vi "Test Filter.vi"() -> ()   [LabVIEW 2021]
uses:
  <vilib>/CIF Foundation/CIF Enet Parse and Build/typedef/L2 & L3/L2-L3 Packet  Addressing.ctl
  <vilib>/CIF Foundation/CIF Enet Parse and Build/typedef/L2 & L3/Packet Type.ctl
  <vilib>/CIF Foundation/CIF Enet Parse and Build/typedef/L2 & L3/IPV4 Filter.ctl
  <vilib>/CIF Foundation/CIF Enet Parse and Build/typedef/L2 & L3/IPV4 Protocol Ring.ctl
  <vilib>/CIF Foundation/CIF Enet Parse and Build/typedef/L2 & L3/L2 Filter.ctl
  L2ENET_RW_XNET/src/typedef/trash_Filter.ctl
  L2ENET_RW_CORE.lvclass/L2ENET_RW_CORE.ctl
  Accessors/Write Filter.vi
  <vilib>/CIF Foundation/CIF Utilities/Networking/IPV4/Calculate IP Header Checksum.vi
  <vilib>/CIF Foundation/CIF Enet Parse and Build/Packet Parse and Build/Packet Create L2&L3/Worker SubVIs/Create UDP Pseudoheader.vi
  <vilib>/CIF Foundation/CIF Enet Parse and Build/Packet Parse and Build/Packet Create L2&L3/Create UDP Header.vi
  <vilib>/CIF Foundation/CIF Enet Parse and Build/Packet Parse and Build/Packet Create L2&L3/Create IPV4 Header.vi
  <vilib>/CIF Foundation/CIF Enet Parse and Build/Packet Parse and Build/Packet Create L2&L3/Create L2 Header.vi
  <vilib>/CIF Foundation/CIF Enet Parse and Build/Packet Parse and Build/Filter and Parse L2&L3/Filter.vi
  <vilib>/CIF Foundation/CIF Utilities/DataTypes/Flatten Unflatten/Flatten U32.vi
  <vilib>/CIF Foundation/CIF Utilities/DataTypes/Flatten Unflatten/Flatten U16.vi
  <vilib>/CIF Foundation/CIF Utilities/DataTypes/Split Join/Join U8.vi
  <vilib>/CIF Foundation/CIF Utilities/DataTypes/Split Join/Join U16.vi
  <vilib>/CIF Foundation/CIF Enet Parse and Build/Packet Parse and Build/Packet Create L2&L3/Worker SubVIs/Create VLAN Tag.vi
  <vilib>/CIF Foundation/CIF Enet Parse and Build/Packet Parse and Build/Utilities/Create Multicast MAC Address.vi
  <vilib>/CIF Foundation/CIF Utilities/Networking/IPV4/Check Multicast IP.vi
  <vilib>/CIF Foundation/CIF Enet Parse and Build/Packet Parse and Build/Filter and Parse L2&L3/Parse L2 Header.vi
  <vilib>/CIF Foundation/CIF Enet Parse and Build/Packet Parse and Build/Filter and Parse L2&L3/Parse IPV4 Header.vi
  <vilib>/CIF Foundation/CIF Enet Parse and Build/Packet Parse and Build/Filter and Parse L2&L3/Parse UDP Header.vi
  <vilib>/CIF Foundation/CIF Enet Parse and Build/Packet Parse and Build/Filter and Parse L2&L3/Parse TCP Header.vi
  <vilib>/CIF Foundation/CIF Utilities/DataTypes/Flatten Unflatten/Unflatten U16.vi
  <vilib>/CIF Foundation/CIF Utilities/DataTypes/Split Join/Split U8.vi
  <vilib>/CIF Foundation/CIF Utilities/DataTypes/Flatten Unflatten/Unflatten U32.vi
  <vilib>/CIF Foundation/CIF Utilities/DataTypes/Split Join/Split U16.vi
  L2ENET_RW_CORE.lvclass
  <vilib>/CIF Foundation/CIF Enet Parse and Build/Ethernet_Parse_Build_CIF.lvlib
panel:
  out "Pass":bool
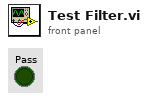
[diagram p1: front panel]
types:
  T1 = typedef "trash_Filter.ctl" = cluster{"L2 Filter":T2, "IPV4 Filter":T3}
  T2 = typedef "Ethernet_Parse_Build_CIF.lvlib/L2 Filter.ctl" = cluster{"DMAC Filter":bool, "DMAC":u8[], "SMAC Filter":bool, "SMAC":u8[], "EtherType Filter":bool, "EtherType":u16, "VLAN Filter":bool, "VLAN":u16, "PCP Filter":bool, "PCP":u8}
  T3 = typedef "Ethernet_Parse_Build_CIF.lvlib/IPV4 Filter.ctl" = cluster{"Source IP Filter":bool, "Source IP Address":u32, "Destination  IP Filter":bool, "Dest IP Address":u32, "IP Protocol Filter":bool, "Protocol":T4, "Source Port Filter":bool, "Source Port":u16, "Dest Port Filter ":bool, "Dest Port":u16}
  T4 = typedef "Ethernet_Parse_Build_CIF.lvlib/IPV4 Protocol Ring.ctl" = u8
  T5 = typedef "Ethernet_Parse_Build_CIF.lvlib/L2-L3 Packet  Addressing.ctl" = cluster{"Dest MAC Address":u8[], "Source MAC Address":u8[], "Packet Type":T6, "Ethertype":u16, "Source IP Address":u32, "Dest IP Address":u32, "DST Port":u16, "SRC Port":u16, "VLAN Tagged?":bool, "VLAN":u16, "PCP":u8}
  T6 = typedef "Ethernet_Parse_Build_CIF.lvlib/Packet Type.ctl" = enum16{"RAW", "UDP"}
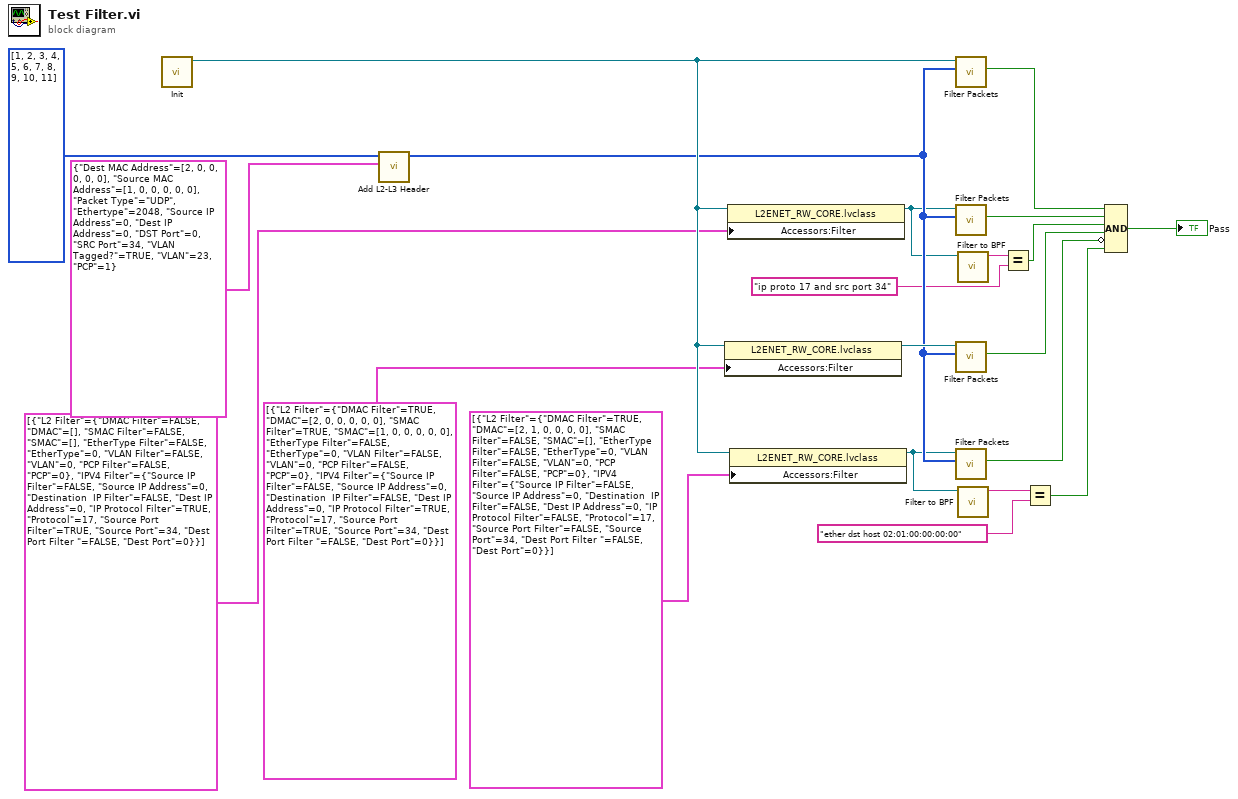
[diagram p0: block diagram]
diagram:
  n1 = call "Init.vi"() -> ("L2Enet_RW_CORE out"=w19:refnum<class "L2ENET_RW_CORE.lvclass">)  [unwired: 10 in, 1 out]
  n2 = call <vilib>:"Add L2-L3 Header.vi"("Addressing"=T5 {"Dest MAC Address"=[2, 0, 0, 0, 0, 0], "Source MAC Address"=[1, 0, 0, 0, 0, 0], "Packet Type"=enum."UDP", "Ethertype"=2048, "Source IP Address"=0, "Dest IP Address"=0, "DST Port"=0, "SRC Port"=34, "VLAN Tagged?"=TRUE, "VLAN"=23, "PCP"=1}, "Payload (bytes)"=u8[] [1, 2, 3, 4, 5, 6, 7, 8, 9, 10, 11]) -> ("Packet Data Out"=w12:u8[])  [unwired: 9 in]
  n3 = property class="L2ENET_RW_CORE.lvclass"(reference=w19, "Accessors:Filter"=T1[] [{"L2 Filter"={"DMAC Filter"=TRUE, "DMAC"=[2, 0, 0, 0, 0, 0], "SMAC Filter"=TRUE, "SMAC"=[1, 0, 0, 0, 0, 0], "EtherType Filter"=FALSE, "EtherType"=0, "VLAN Filter"=FALSE, "VLAN"=0, "PCP Filter"=FALSE, "PCP"=0}, "IPV4 Filter"={"Source IP Filter"=FALSE, "Source IP Address"=0, "Destination  IP Filter"=FALSE, "Dest IP Address"=0, "IP Protocol Filter"=TRUE, "Protocol"=17, "Source Port Filter"=TRUE, "Source Port"=34, "Dest Port Filter "=FALSE, "Dest Port"=0}}] ("Filter")) -> (reference out=w18:refnum<class "L2ENET_RW_CORE.lvclass">)  [unwired: 1 in, 1 out]
  n4 = property class="L2ENET_RW_CORE.lvclass"(reference=w19, "Accessors:Filter"=T1[] [{"L2 Filter"={"DMAC Filter"=FALSE, "DMAC"=[], "SMAC Filter"=FALSE, "SMAC"=[], "EtherType Filter"=FALSE, "EtherType"=0, "VLAN Filter"=FALSE, "VLAN"=0, "PCP Filter"=FALSE, "PCP"=0}, "IPV4 Filter"={"Source IP Filter"=FALSE, "Source IP Address"=0, "Destination  IP Filter"=FALSE, "Dest IP Address"=0, "IP Protocol Filter"=TRUE, "Protocol"=17, "Source Port Filter"=TRUE, "Source Port"=34, "Dest Port Filter "=FALSE, "Dest Port"=0}}] ("Filter")) -> (reference out=w8:refnum<class "L2ENET_RW_CORE.lvclass">)  [unwired: 1 in, 1 out]
  n5 = property class="L2ENET_RW_CORE.lvclass"(reference=w19, "Accessors:Filter"=T1[] [{"L2 Filter"={"DMAC Filter"=TRUE, "DMAC"=[2, 1, 0, 0, 0, 0], "SMAC Filter"=FALSE, "SMAC"=[], "EtherType Filter"=FALSE, "EtherType"=0, "VLAN Filter"=FALSE, "VLAN"=0, "PCP Filter"=FALSE, "PCP"=0}, "IPV4 Filter"={"Source IP Filter"=FALSE, "Source IP Address"=0, "Destination  IP Filter"=FALSE, "Dest IP Address"=0, "IP Protocol Filter"=FALSE, "Protocol"=17, "Source Port Filter"=FALSE, "Source Port"=34, "Dest Port Filter "=FALSE, "Dest Port"=0}}] ("Filter")) -> (reference out=w11:refnum<class "L2ENET_RW_CORE.lvclass">)  [unwired: 1 in, 1 out]
  n6 = call "Filter Packets.vi"("L2 Packet in"=w12, "L2Enet_RW_CORE"=w19) -> ("Valid"=w14:bool)  [unwired: 9 in]
  n7 = call "Filter Packets.vi"("L2 Packet in"=w12, "L2Enet_RW_CORE"=w8) -> ("Valid"=w17:bool)  [unwired: 9 in]
  n8 = call "Filter Packets.vi"("L2 Packet in"=w12, "L2Enet_RW_CORE"=w18) -> ("Valid"=w16:bool)  [unwired: 9 in]
  n9 = call "Filter Packets.vi"("L2 Packet in"=w12, "L2Enet_RW_CORE"=w11) -> ("Valid"=w15:bool)  [unwired: 9 in]
  n10 = call "Filter to BPF.vi"("L2ENET_RW_CORE in"=w8) -> ("BPF Format"=w7:string)  [unwired: 9 in, 1 out]
  n11 = call "Filter to BPF.vi"("L2ENET_RW_CORE in"=w11) -> ("BPF Format"=w10:string)  [unwired: 9 in, 1 out]
  n12 = Equal?(x=w7, y="ip proto 17 and src port 34" ("BPF Format")) -> (x = y?=w5:bool)
  n13 = Equal?(x=w10, y="ether dst host 02:01:00:00:00:00" ("BPF Format")) -> (x = y?=w4:bool)
  n14 = Compound Arithmetic op=AND(w14, w17, w5, w16, invert w15, w4) -> (→"Pass":bool)
